vi "Header.vi"(0 "Consumer P/N":string, 3 "GeneralResult":string, 5 "P/N UUT":string, 9 "Driver S/N":string, 11 "error in":errorcluster, 12 "ParametersVer":string, 13 "Oper.":string, 14 "Tester Software Ver":string) -> (6 "Array":string[][](array[string]), 15 "error out":errorcluster)   [LabVIEW 2017]
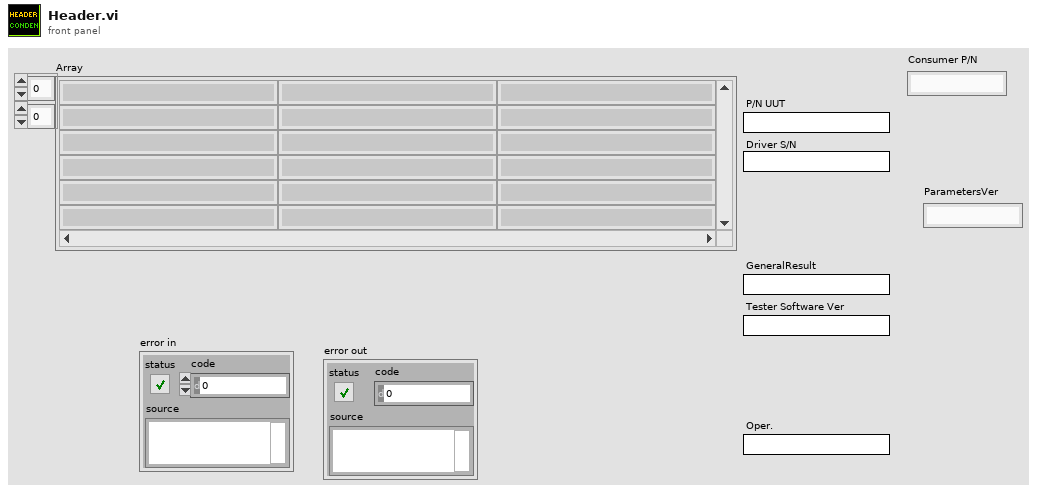
[diagram p1: front panel]
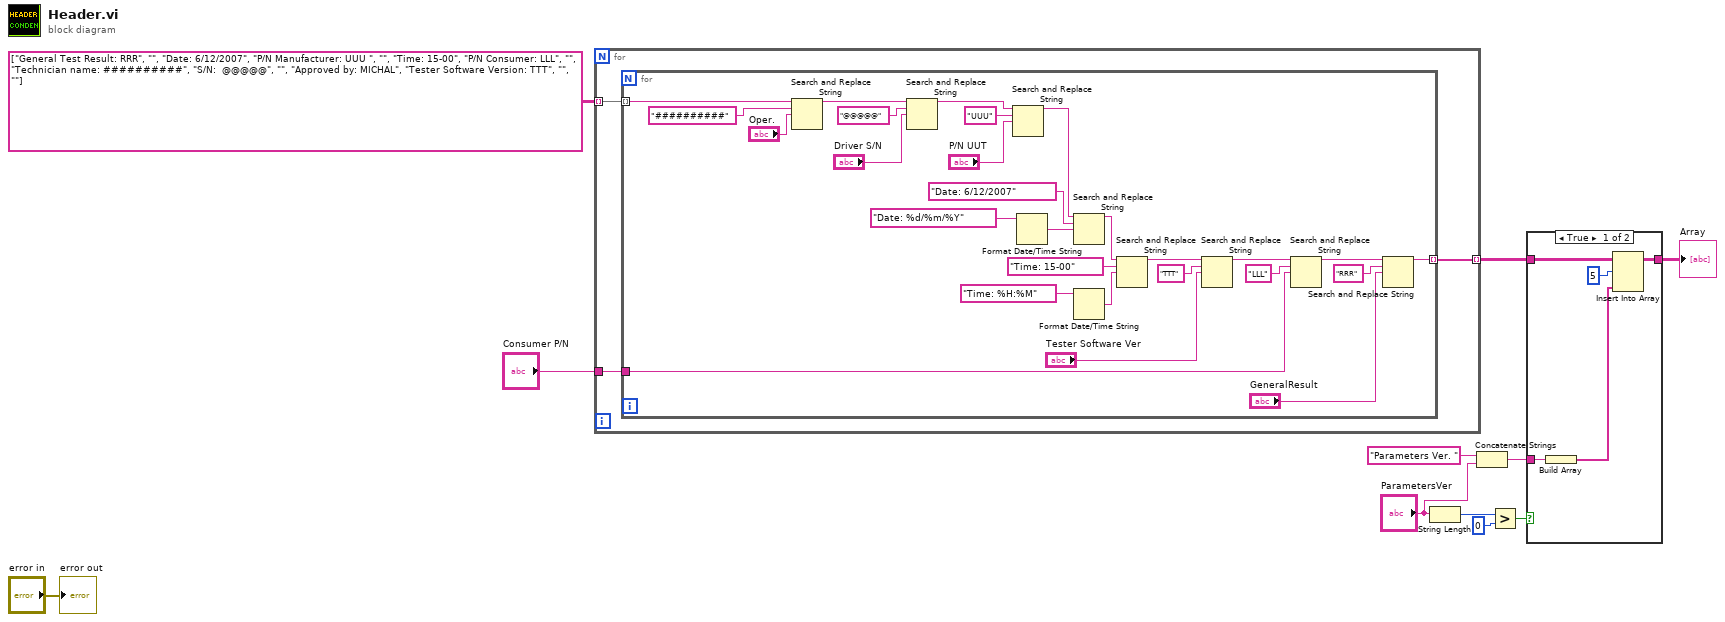
[diagram p0: block diagram]
diagram:
  n1 = for {
    tunnel: string[][] [["General Test Result: RRR", "", "Date: 6/12/2007"], ["P/N Manufacturer: UUU ", "", "Time: 15-00"], ["P/N Consumer: LLL", "", "Technician name: ##########"], ["S/N:  @@@@@", "", "Approved by: MICHAL"], ["Tester Software Version: TTT", "", ""]] -> [w14] mode=indexing
    tunnel: [w13] -> w6 mode=indexing
    tunnel: "Consumer P/N" -> [w12]
    n2 = for {
      tunnel: w14 -> [w20] mode=indexing
      tunnel: [w19] -> w13 mode=indexing
      tunnel: w12 -> [w15]
      n3 = Search and Replace String(input string=w20, search string="##########" ("source"), replace string="Oper.") -> (result string=w31:string)  [unwired: 5 in, 3 out]
      n4 = Search and Replace String(input string=w31, search string="@@@@@" ("source"), replace string="Driver S/N") -> (result string=w33:string)  [unwired: 5 in, 3 out]
      n5 = Search and Replace String(input string=w33, search string="UUU" ("source"), replace string="P/N UUT") -> (result string=w32:string)  [unwired: 5 in, 3 out]
      n6 = Format Date/Time String(time format string (%c)="Date: %d/%m/%Y") -> (date/time string=w30:string)  [unwired: 2 in]
      n7 = Search and Replace String(input string=w32, search string="Date: 6/12/2007" ("time format string (%c)"), replace string=w30) -> (result string=w38:string)  [unwired: 5 in, 3 out]
      n8 = Format Date/Time String(time format string (%c)="Time: %H:%M") -> (date/time string=w40:string)  [unwired: 2 in]
      n9 = Search and Replace String(input string=w38, search string="Time: 15-00", replace string=w40) -> (result string=w39:string)  [unwired: 5 in, 3 out]
      n10 = Search and Replace String(input string=w39, search string="TTT", replace string="Tester Software Ver") -> (result string=w18:string)  [unwired: 5 in, 3 out]
      n11 = Search and Replace String(input string=w18, search string="LLL", replace string=w15) -> (result string=w17:string)  [unwired: 5 in, 3 out]
      n12 = Search and Replace String(input string=w17, search string="RRR", replace string="GeneralResult") -> (result string=w19:string)  [unwired: 5 in, 3 out]
    }
  }
  n13 = String Length(string="ParametersVer") -> (length=w3:i32)
  n14 = Concatenate Strings("Parameters Ver. " ("string"), "ParametersVer") -> (w4:string)
  n15 = Greater?(x=w3, y=0) -> (0:w1:bool)
  n16 = case shown="True" w1 {
    tunnel: w6 -> [w46 w47]
    tunnel: [w42 w47] -> w5
    tunnel: w4 -> [w44 _]
    frame True {
      n17 = Build Array(w44) -> (w43:string[])
      n18 = Insert Into Array(array=w46, index (row)=5, new element=w43) -> (w42:string[][])  [unwired: 1 in]
    }
    frame False {
    }
  }
  "Array" <- w5
  "error out" <- "error in"
